vi "GenericDAQCore.vi"(8 "error in":errorcluster, 9 "SignalBuffer queue in":refnum<queue>, 10 "GenericDAQ CtrlQueue in":refnum<queue>) -> (0 "error out":errorcluster)   [LabVIEW 2014, in "GenericDAQ.lvlib"]
uses:
  <instrlib>/GenericDAQ/GenericDAQ.lvlib
  <instrlib>/GenericDAQ/VI/GenericDAQ_Ctrl_Queue.ctl
  <instrlib>/GenericDAQ/VI/GenericDAQ_State.ctl
  <instrlib>/GenericDAQ/VI/GenericDAQ_Signal.ctl
  <instrlib>/GenericDAQ/VI/GenericDAQ_Configs.ctl
  <instrlib>/GenericDAQ/VI/GenericDAQ_PrivateStats.ctl
  <instrlib>/GenericDAQ/VI/GenericDAQ_Status.ctl
  <vilib>/Utility/error.llb/DialogType.ctl
  <instrlib>/GageLv_uic/VI/SetSecondaryDataVIRef_Typedef.ctl
  <vilib>/Utility/error.llb/Error Cluster From Error Code.vi
  <instrlib>/GenericDAQ/VI/InstrParams.vi
  <vilib>/ErrorRing/Error Ring.xnode
  <userlib>/Utility/ErrorLog_lib.lvlib
panel:
  in  "StartAll":bool
  out "Core#":i32
  in  "Get_ConfigAll":bool
  out "LiveStat":T1
  in  "GenericDAQ_Config":T3={"Acquisition"={"Sample Rate"=1000000000.0, "Mode"=0, "Start (0)"=0.0, "Depth"=8192.0, "Segment"=1}, "Channels"=[{"Range"=1, "DC Offset"=0}], "Mode(Gage)"=enum."Continuous"} {"Acquisition"."Depth" min=256.0 step=128.0; "Acquisition"."Mode" items=["Single", "Dual", "Quad", "Octal"]; "Acquisition"."Sample Rate" format="%.0p"}
  out "Graph":sgl[](graph)
  in  "fConfig":bool
  in  "Reset":bool
  in  "CloseAll":bool
  in  "Close":bool
  in  "Enumerate":bool
  in  "Open":bool
  in  "Quit":bool
  in  "Start":bool
  in  "ConfigAll":bool
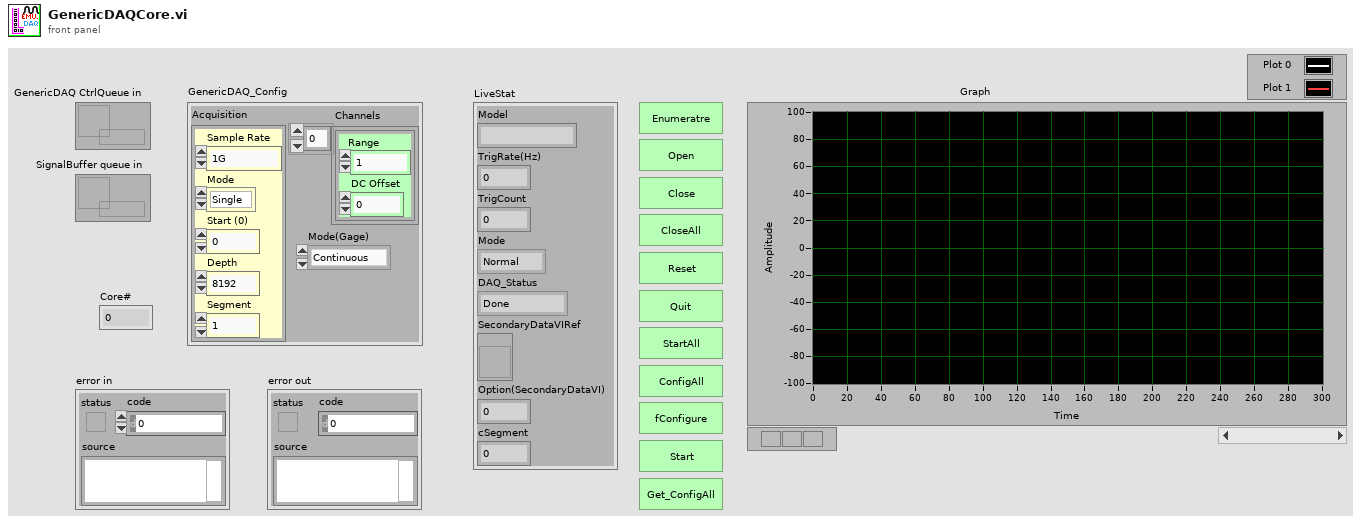
[diagram p1: front panel]
types:
  T1 = typedef "GenericDAQ.lvlib/GenericDAQ_PrivateStats.ctl" = cluster{"Model":string, "TrigRate(Hz)":dbl, "TrigCount":i32, "Mode":enum16{"Normal", "Continuous", "MultiRecord", "HwAverage"}, "DAQ_Status":T2, "SecondaryDataVIRef":refnum<vi>, "Option(SecondaryDataVI)":i32, "cSegment":i32}
  T2 = typedef "GenericDAQ.lvlib/GenericDAQ_Status.ctl" = enum16{"Done", "Armed", "Triggered", "Transfering"}
  T3 = typedef "GenericDAQ.lvlib/GenericDAQ_Configs.ctl" = cluster{"Acquisition":cluster{"Sample Rate":dbl, "Mode":u16, "Start (0)":dbl, "Depth":dbl, "Segment":u32}, "Channels":cluster{"Range":u32, "DC Offset":i32}[], "Mode(Gage)":enum16{"Normal", "Continuous", "MultiRecord", "HwAverage"}}
  T4 = enum16{"Normal", "MultiRecStart", "MultiRecEnd", "Reserved1", "Reserved2", "Reserved3"}
  T5 = typedef "DialogType.ctl" = u16
  T6 = typedef "GenericDAQ.lvlib/GenericDAQ_Signal.ctl" = cluster{"tickcount":u32, "Signal":sgl[], "SecondaryData":dbl[], "Flag":enum16{"Normal", "LineStart", "LineEnd", "FrameStart", "FrameEnd", "Reserved1", "Reserved2"}, "Segment#":i32}
  T7 = enum16{"Normal", "Continuous", "MultiRecord", "HwAverage"}
  T8 = typedef "GenericDAQ.lvlib/GenericDAQ_Ctrl_Queue.ctl" = cluster{"GenericDAQ State":T9, "Variant":variant}
  T9 = typedef "GenericDAQ.lvlib/GenericDAQ_State.ctl" = enum16{"Enumerate", "Open", "Close", "CloseAll", "Reset", "Quit", "==Settings==", "SetAcquisition_", "SetChannels_", "SetTrigger_", "SetAnalogTrigDetector_", "SetSegment#_", "SetAll_AcquChTrig_", "fConfigurate", "fStart", "GetStatus", "_WaitForDone/Idle", "_GetData", "GetAcquisition", "GetChannels", "GetTrigger", "GetAll_AcquChTrig", "Abort", "==Messaging==", "_PushDataOut", "GetStat_", "GetConfig_", "==ModeSetup==", "SetSignalBuffer_", "SetMode_", "SetSecondaryDataRef._", "SetDynamicBuffer_", "==AnalogOut==", "GetChannelCount_AO", "fStart_AO", "SetChEnable_AO", "SetConfig_AO", "SetFuncData_AO", "SetOffset_AO_", "SetMasterNode_AO", "SetStates_AO", "SetSymetry_AO", "SetTriggerSource_AO", "==Trigger==", "ManualTrigger", "===Sync===", "LineStart", "LineEnd", "FrameStart", "FrameEnd", "EOL_PassThrough", "SOL_PassThrough"}
  T10 = typedef "SetSecondaryDataVIRef_Typedef.ctl" = cluster{"SecondaryDataVIRef.":refnum<vi>, "Option":i32}
  T11 = cluster{"Handle":u32, "Sample size":u32, "Resolution":i32, "Offset":i32, "Channels":u32, "Boards":u32}
  T12 = cluster{"Sample Rate":dbl, "Mode":u16, "Start (0)":dbl, "Depth":dbl, "Segment":u32}
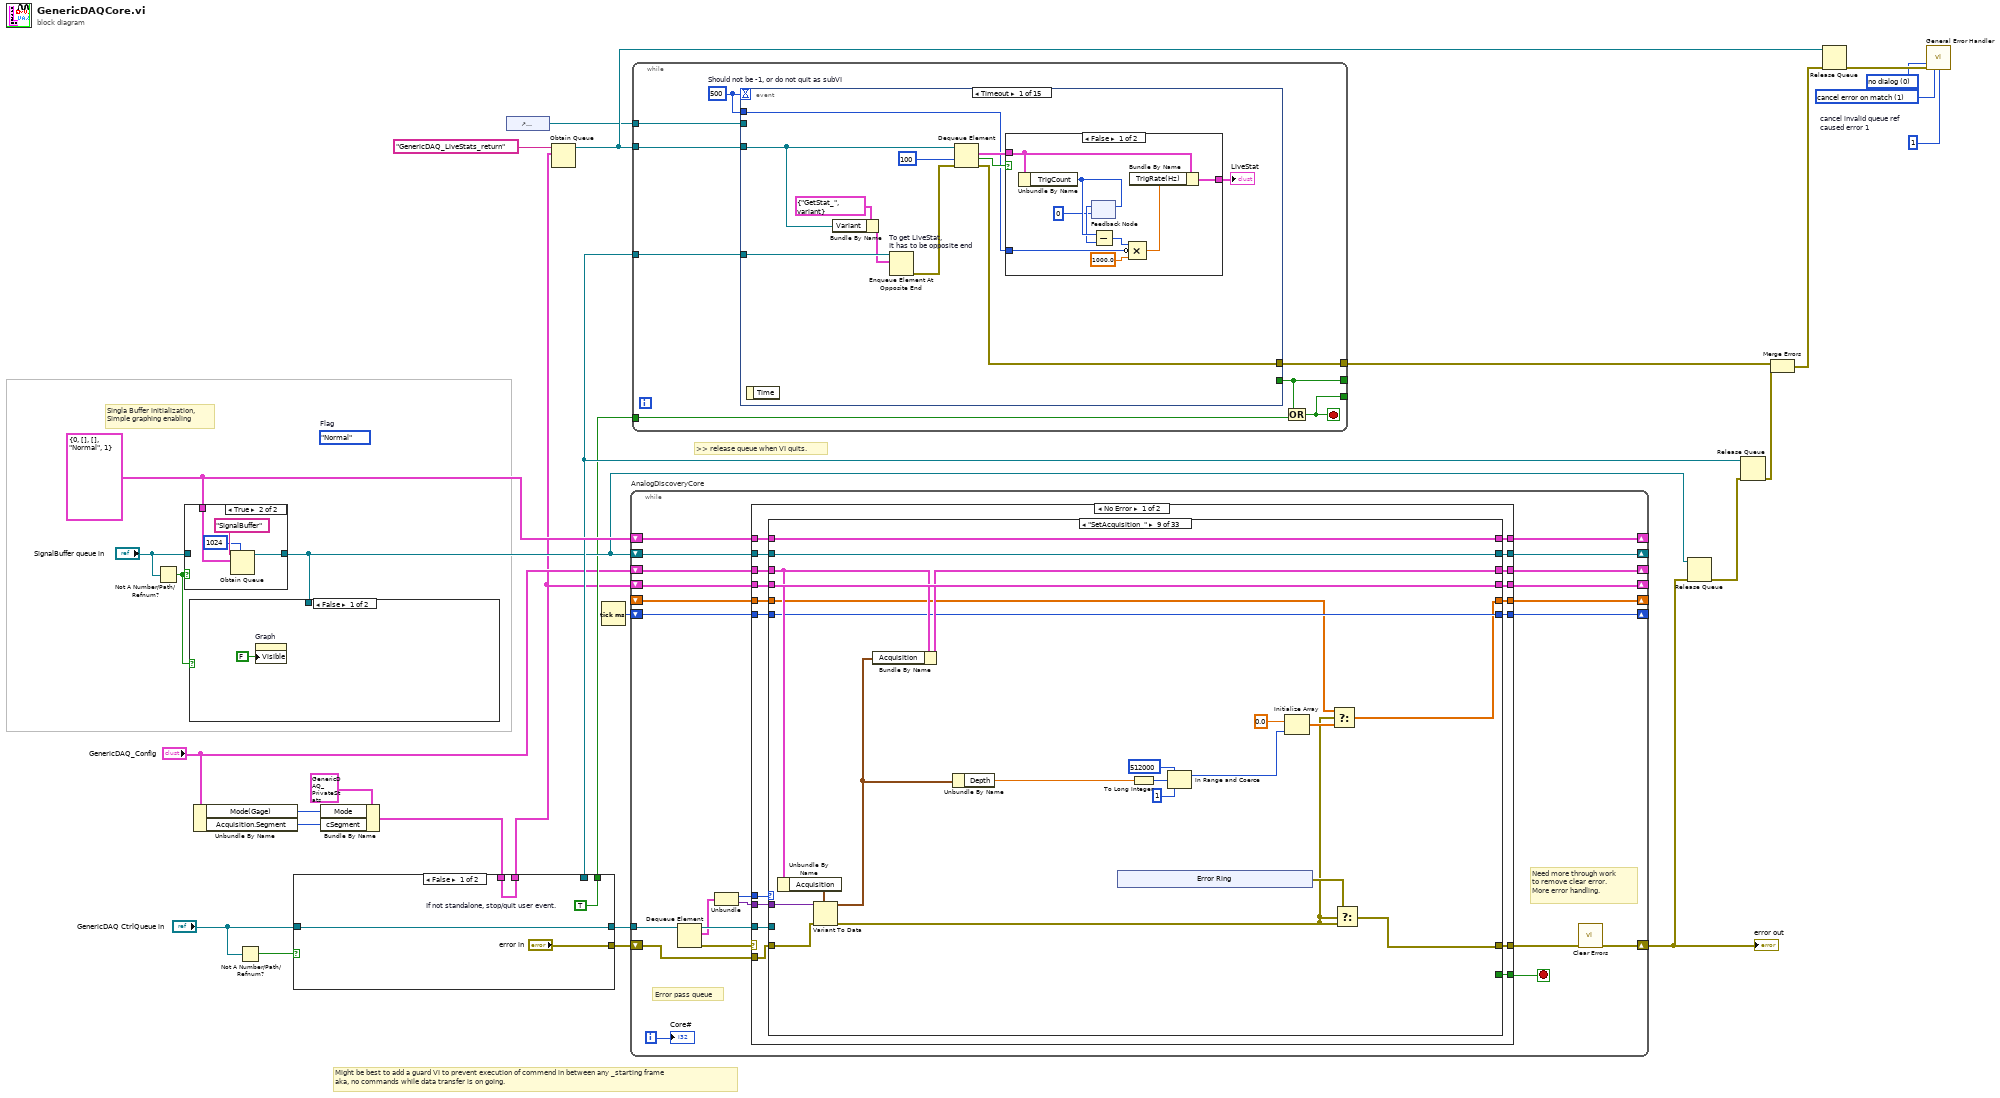
[diagram p0: block diagram]
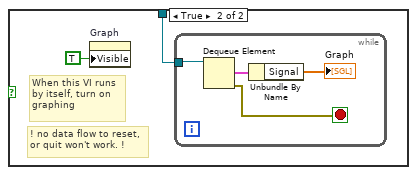
[diagram p2: hidden frame]
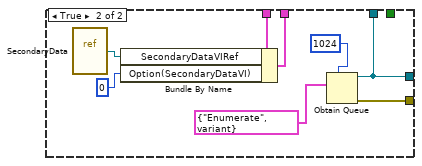
[diagram p4: hidden frame]
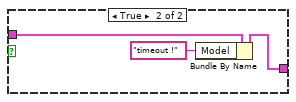
[diagram p5: hidden frame]
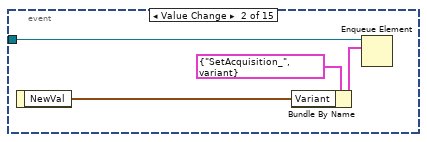
[diagram p6: hidden frame]
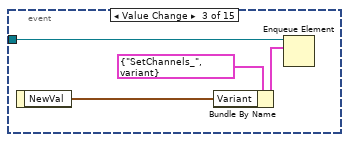
[diagram p7: hidden frame]
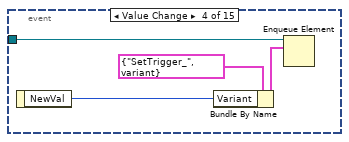
[diagram p8: hidden frame]
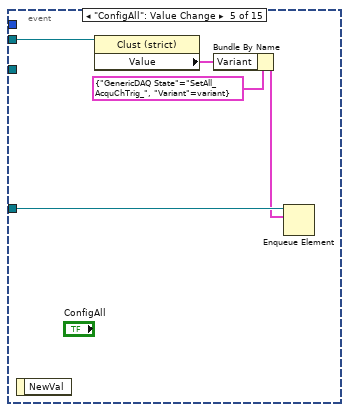
[diagram p9: hidden frame]
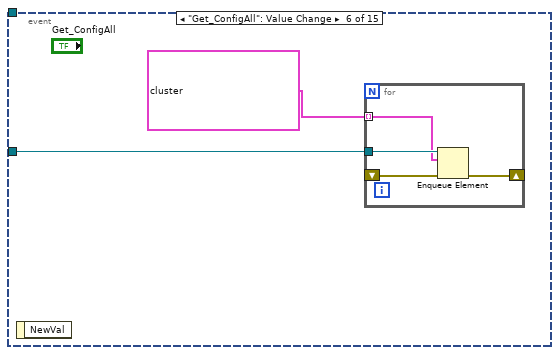
[diagram p10: hidden frame]
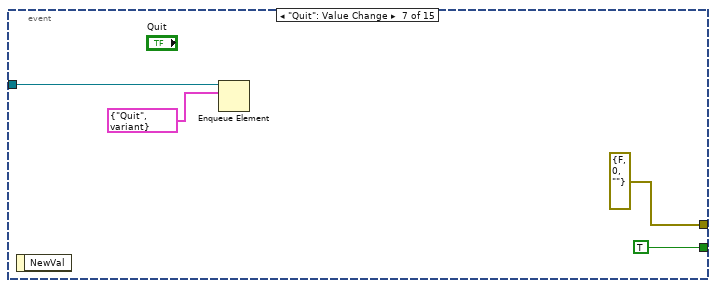
[diagram p11: hidden frame]
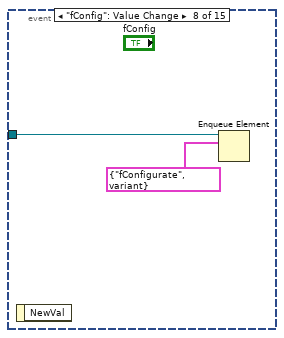
[diagram p12: hidden frame]
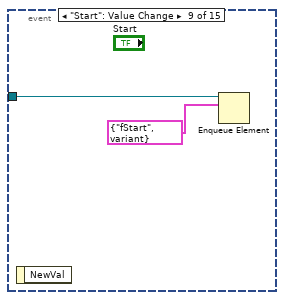
[diagram p13: hidden frame]
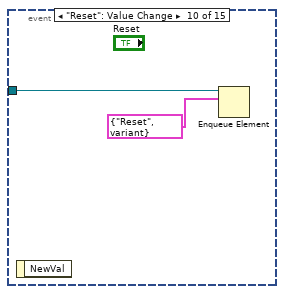
[diagram p14: hidden frame]
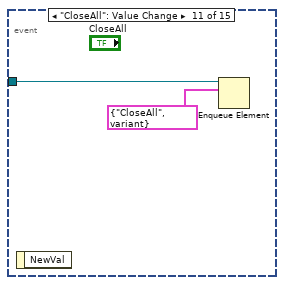
[diagram p15: hidden frame]
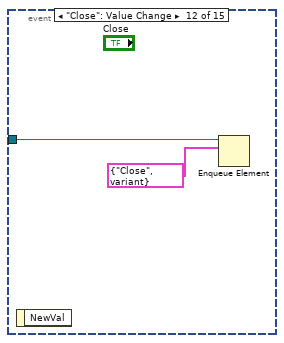
[diagram p16: hidden frame]
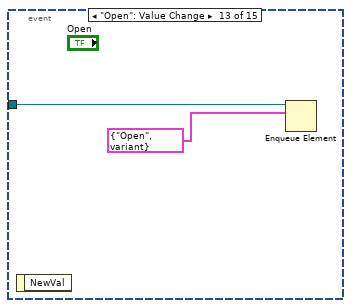
[diagram p17: hidden frame]
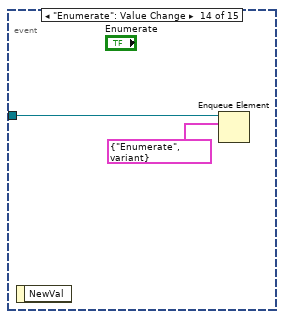
[diagram p18: hidden frame]
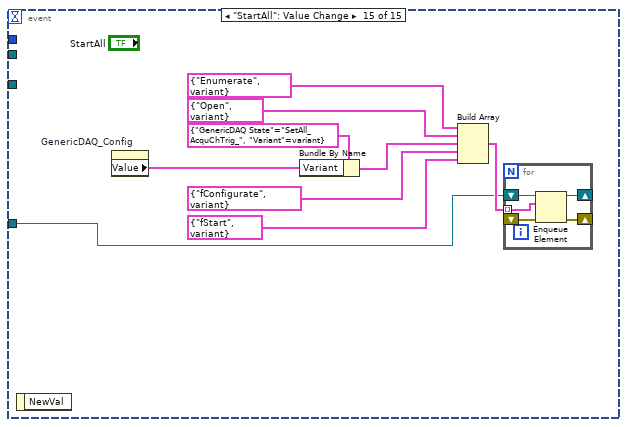
[diagram p19: hidden frame]
diagram:
  (unwired) T4."Normal"  # Flag
  w11 = 1  # cancel invalid queue ref caused error 1
  w12 = 1 items=["no exception", "cancel error on match", "set error on match"] ("[exception action] (none:0)")
  w13 = T5 0 items=["no dialog", "OK message", "continue or stop message", "OK message + warnings", "continue/stop + warnings"] ("type of dialog (OK msg:1)")
  w29 = T6 {"tickcount"=0, "Signal"=[], "SecondaryData"=[], "Flag"=enum."Normal", "Segment#"=1} ("Signal_Typedef")
  # "Might be best to add a guard VI to prevent execution of commend in between any _starting frame \naka, no commands while data transfer is on going."
  # "Singla Buffer initialization,\nSimple graphing enabling"
  # ">> release queue when VI quits."
  n1 = Not A Number/Path/Refnum?(number/path/refnum="SignalBuffer queue in") -> (NaN/Path/Refnum?=w16:bool)
  n2 = case shown="True" w16 {
    tunnel: w29 -> [_ w34]
    tunnel: [w30 w31] -> w17
    tunnel: "SignalBuffer queue in" -> [w30 _]
    frame False {
    }
    frame True {
      n3 = Obtain Queue(max queue size (-1, unlimited)=1024, name (unnamed)="SignalBuffer", element data type=w34) -> (queue out=w31:refnum<queue>)  [unwired: 2 in, 2 out]
    }
  }
  n4 = case shown="False" w16 {
    tunnel: w17 -> [_ w37]
    frame False {
      n5 = property on="Graph" class="WFGraph (strict)"("Visible"=FALSE) -> ()  [unwired: 2 in, 2 out]
    }
    frame True {
      # "! no data flow to reset,\nor quit won't work. !"
      # "When this VI runs\nby itself, turn on \ngraphing"
      n6 = property on="Graph" class="WFGraph (strict)"("Visible"=TRUE) -> ()  [unwired: 2 in, 2 out]
      n7 = while {
        tunnel: w37 -> [w41]
        stop <- w38 stop-if-true
        n8 = Dequeue Element(queue=w41) -> (element=w40:T6, error out=w38:errorcluster)  [unwired: 2 in, 2 out]
        n9 = Unbundle By Name(w40) -> ("Signal"=→"Graph":sgl[])
      }
    }
  }
  n10 = Unbundle By Name("GenericDAQ_Config") -> ("Mode(Gage)"=w7:T7, "Acquisition.Segment"=w4:u32)
  n11 = Not A Number/Path/Refnum?(number/path/refnum="GenericDAQ CtrlQueue in") -> (NaN/Path/Refnum?=w26:bool)
  n12 = Bundle By Name(cluster=T1 {"Model"="", "TrigRate(Hz)"=0.0, "TrigCount"=0, "Mode"=enum."Normal", "DAQ_Status"=enum."Done", "SecondaryDataVIRef"=refnum, "Option(SecondaryDataVI)"=0, "cSegment"=0} ("PrivateStats(Live)"), "Mode"=w7, "cSegment"=w4) -> (w1:T1)
  n13 = case shown="False" w26 {
    tunnel: [w45 w50] -> w28
    tunnel: ["error in" w53] -> w27
    tunnel: "GenericDAQ CtrlQueue in" -> [w45 _]
    tunnel: [_ w50] -> w22
    tunnel: [w43 _] -> w10
    tunnel: [w42 w47] -> w2
    tunnel: w1 -> [w42 w46]
    frame False {
      w43 = TRUE  # If not standalone, stop/quit user event.
    }
    frame True {
      n14 = vi-ref <instrlib>:"SecondaryData.vi"() -> (w49:refnum<vi>)
      n15 = Bundle By Name(cluster=w46, "SecondaryDataVIRef"=w49, "Option(SecondaryDataVI)"=0) -> (w47:T1)
      n16 = Obtain Queue(max queue size (-1, unlimited)=1024, element data type=T8 {"GenericDAQ State"=enum."Enumerate", "Variant"=variant}) -> (queue out=w50:refnum<queue>, error out=w53:errorcluster)  [unwired: 3 in, 1 out]
    }
  }
  n17 = control-ref of="GenericDAQ_Config"() -> (w5:refnum<vi>)
  n18 = Obtain Queue(name (unnamed)="GenericDAQ_LiveStats_return", element data type=w2) -> (queue out=w20:refnum<queue>)  [unwired: 3 in, 2 out]
  n19 = Tick Count (ms)() -> (millisecond timer value=w3:u32)
  n20 = while "AnalogDiscoveryCore" {
    shift-right: [w75] -> _
    shift-left: w17 -> [w76]
    tunnel: w28 -> [w62]
    shift-right: [w56] -> w15
    shift-left: w27 -> [w64]
    shift-right: [w73] -> _
    shift-left: "GenericDAQ_Config" -> [w72]
    shift-right: [w60] -> _
    shift-left: w2 -> [w71]
    shift-right: [w65] -> _
    shift-left: _ -> [w69]
    shift-right: [w66] -> _
    shift-left: w29 -> [w70]
    shift-right: [w54] -> _
    shift-left: w3 -> [w55]
    i -> [w58]
    stop <- w74 stop-if-true
    # "Need more through work\nto remove clear error.\nMore error handling."
    # "Error pass queue"
    n21 = Dequeue Element(queue=w62) -> (queue out=w61:refnum<queue>, element=w59:T8, error out=w63:errorcluster)  [unwired: 2 in, 1 out]
    n22 = Unbundle(w59) -> ("GenericDAQ State"=w68:T9, "Variant"=w67:variant)
    n23 = case shown="No Error" w63 {
      tunnel: w76 -> [w94 w727]
      tunnel: [w93 w727] -> w75
      tunnel: [w92 TRUE] -> w74
      tunnel: [w91 w725] -> w57
      tunnel: [w90 w728] -> w73
      tunnel: w72 -> [w89 w728]
      tunnel: w71 -> [w88 w729]
      tunnel: w70 -> [w87 w726]
      tunnel: w69 -> [w86 w730]
      tunnel: w61 -> [w85 _]
      tunnel: w68 -> [w84 _]
      tunnel: w67 -> [w83 _]
      tunnel: [w82 w726] -> w66
      tunnel: [w81 w730] -> w65
      tunnel: [w80 w729] -> w60
      tunnel: w64 -> [w79 _]
      tunnel: w55 -> [w78 w724]
      tunnel: [w77 w724] -> w54
      frame No Error {
        n24 = case shown="\"SetAcquisition_\"" w84 {
          tunnel: w94 -> [w101 w108 w132 w139 w146 w160 w172 w179 w206 w224 w245 w257 w297 w328 w362 w393 w443 w495 w504 w511 w521 w532 w555 w593 w605 w618 w630 w654 w666 w691 w707 w708 w716]
          tunnel: [w101 w108 w132 w139 w146 w160 w172 w179 w206 w224 w245 w257 w297 w328 w362 w393 w443 w495 w504 w511 w521 w532 w555 w593 w605 w618 w631 w654 w666 w690 w707 w708 w716] -> w93
          tunnel: [_ _ _ _ _ _ TRUE _ _ _ _ _ _ _ _ _ _ _ _ _ _ _ _ _ _ _ _ _ _ _ _ _ _] -> w92
          tunnel: w85 -> [_ _ _ _ _ w156 _ _ _ _ _ w254 w287 w322 _ w395 w439 _ _ _ w516 _ w551 _ _ _ _ _ _ _ _ _ _]
          tunnel: w79 -> [w100 w104 w128 w134 w145 w155 w167 _ w198 w215 _ w248 w288 w319 w358 w394 w437 w494 w503 w510 w515 _ w553 w587 w597 _ w627 w644 _ w694 w706 w715 w723]
          tunnel: [w100 w104 errorcluster {"status"=FALSE, "code"=0, "source"=""} ("error out") w134 w145 w154 w167 w174 w185 w216 errorcluster {"status"=FALSE, "code"=0, "source"=""} ("error out") w253 w286 w323 w358 w388 w440 w494 w503 w510 w514 w527 w552 w586 w598 w613 w628 w645 w656 w694 w706 w715 w723] -> w91
          tunnel: [w99 w107 w131 w138 w144 w159 w171 w178 w203 w221 w241 w251 w296 w327 w361 w392 w445 w490 w500 w509 w517 w531 w549 w585 w595 w617 w636 w653 w665 w700 w705 w714 w722] -> w90
          tunnel: w89 -> [w99 w107 w131 w138 w144 w159 w171 w178 w201 w219 w241 w251 w296 w327 w361 w392 w445 w489 w498 w509 w517 w531 w549 w585 w595 w617 w636 w653 w665 w700 w705 w714 w722]
          tunnel: [w98 w106 w124 w136 w141 w153 w168 w177 w204 w222 w243 w247 w294 w325 w357 w385 w419 w491 w499 w506 w520 w530 w547 w584 w604 w616 w635 w650 w662 w699 w704 w713 w721] -> w80
          tunnel: w88 -> [w98 w106 w129 w136 w141 w153 w168 w177 w204 w222 w243 w247 w294 w325 w356 w386 w434 w491 w499 w506 w520 w530 w548 w584 w604 w616 w635 w649 w657 w699 w704 w713 w721]
          tunnel: w87 -> [w97 w105 w130 w137 w143 w158 w170 w176 w205 w223 w244 w256 w295 w326 w360 w391 w442 w493 w502 w508 w519 w529 w541 w592 w603 w615 w634 w652 w664 w698 w703 w712 w720]
          tunnel: w86 -> [w96 w103 _ w135 w142 w157 w169 w175 w188 w213 w242 w255 w293 w321 w359 w387 w444 w492 w501 w507 w518 w528 w539 w591 w602 w614 w633 w651 w663 w697 w702 w711 w719]
          tunnel: w83 -> [_ _ w127 _ _ _ _ _ w202 w220 _ w252 _ _ _ _ _ _ _ _ _ _ _ w588 w601 _ w632 w648 w660 w695 _ _ _]
          tunnel: [w97 w105 w130 w137 w143 w158 w170 w176 w205 w223 w244 w256 w295 w326 w360 w391 w441 w493 w502 w508 w519 w529 w541 w592 w603 w615 w634 w652 w664 w698 w703 w712 w720] -> w82
          tunnel: [w96 w103 w115 w135 w142 w157 w169 w175 w189 w213 w242 w255 w293 w321 w359 w387 w436 w492 w501 w507 w518 w528 w539 w591 w602 w614 w633 w651 w663 w697 w702 w711 w719] -> w81
          tunnel: w78 -> [w95 w102 w109 w133 w140 w149 w166 w173 w196 w212 w239 w246 w285 w314 w344 w367 w417 w487 w496 w505 w513 w526 w538 w582 w596 w612 w624 w642 w655 w696 w701 w710 w718]
          tunnel: [w95 w102 w109 w133 w140 w149 w166 w173 w196 w212 w239 w246 w285 w314 w344 w370 w417 w487 w496 w505 w513 w526 w538 w582 w596 w612 w624 w642 w655 w696 w701 w710 w718] -> w77
          frame Default {
          }
          frame "Enumerate" {
          }
          frame "Open" {
            (unwired) T11 {"Handle"=0, "Sample size"=1, "Resolution"=256, "Offset"=0, "Channels"=0, "Boards"=0} ("Handle")
            w113 = 8192 ("dimension size")
            w114 = 2 ("16KSa, per spec")
            n25 = Variant To Data(error in=w128, type="", Variant=w127) -> (data=w123:string, error out=w125:errorcluster)
            n26 = Select(t="any", s=TRUE, f=w123) -> (s? t:f=w110:string)
            n27 = Wait (ms)(milliseconds to wait=u32 0) -> ()  [unwired: 1 out]
            n28 = Bundle By Name(cluster=w125, "source"=w110) -> ()  [unwired: 1 out]
            n29 = Bundle By Name(cluster=w129, "Model"=w110, "TrigRate(Hz)"=0.0, "TrigCount"=0) -> (w124:T1)
            n30 = Initialize Array(sgl 0.0 ("Numeric"), w113) -> (w115:sgl[])
            n31 = Initialize Array(i16 0 ("Numeric"), w114, w113) -> ()  [unwired: 1 out]
            n32 = Initialize Array(u8 0 ("Numeric"), w114, w113) -> ()  [unwired: 1 out]
          }
          frame "Close" {
          }
          frame "CloseAll" {
          }
          frame "Reset" {
            n33 = Unbundle By Name(w153) -> ("Model"=w152:string)
            n34 = Bundle By Name(cluster=T8 {"GenericDAQ State"=enum."Open", "Variant"=variant} ("element"), "Variant"=w152) -> (w151:T8)
            n35 = Build Array(w151, T8 {"GenericDAQ State"=enum."Close", "Variant"=variant} ("element")) -> (w150:T8[])
            n36 = for {
              tunnel: w156 -> [w164]
              tunnel: w150 -> [w161] mode=indexing
              shift-right: [w162] -> w154
              shift-left: w155 -> [w163]
              n37 = Enqueue Element At Opposite End(queue=w164, element=w161, error in (no error)=w163) -> (error out=w162:errorcluster)  [unwired: 1 in, 2 out]
            }
          }
          frame "Quit" {
          }
          frame "==Settings==" {
            # "Invalid frame"
            n38 = xnode "Error Ring"() -> ("error out"=w174:errorcluster)
          }
          frame "SetAcquisition_" {
            n39 = Unbundle By Name(w201) -> ("Acquisition"=w200:T12)
            n40 = Variant To Data(error in=w198, type=w200, Variant=w202) -> (data=w199:T12, error out=w186:errorcluster)
            n41 = Bundle By Name(cluster=w201, "Acquisition"=w199) -> (w203:T3)
            n42 = Unbundle By Name(w199) -> ("Depth"=w192:dbl)
            n43 = xnode "Error Ring"() -> ("error out"=w187:errorcluster)
            n44 = To Long Integer(number=w192) -> (32bit integer=w191:i32)
            n45 = In Range and Coerce(upper limit=512000, x=w191, lower limit=1) -> (coerced(x)=w190:i32)  [unwired: 1 out]
            n46 = Initialize Array(sgl 0.0 ("Numeric"), w190) -> (w197:sgl[])
            n47 = Select(t=w188, s=w186, f=w197) -> (s? t:f=w189:sgl[])
            n48 = Select(t=w187, s=w186, f=w186) -> (s? t:f=w185:errorcluster)
          }
          frame "SetChannels_" {
            n49 = Unbundle By Name(w219) -> ("Channels"=w218:cluster{"Range":u32, "DC Offset":i32}[])
            n50 = Variant To Data(error in=w215, type=w218, Variant=w220) -> (data=w217:cluster{"Range":u32, "DC Offset":i32}[], error out=w214:errorcluster)
            n51 = Bundle By Name(cluster=w219, "Channels"=w217) -> (w221:T3)
            n52 = case shown="No Error" w214 {
              selector: w214 -> [w225 _]
              tunnel: w222 -> [_ _]
              tunnel: w217 -> [w227 _]
              tunnel: [w226 w233] -> w216
              frame No Error {
                n53 = for {
                  tunnel: w227 -> [w229] mode=indexing
                  shift-right: [w232] -> w226
                  shift-left: w225 -> [w232]
                  tunnel: [w228] -> _ mode=indexing
                  n54 = Unbundle By Name(w229) -> ("Range"=w230:u32, "DC Offset"=w231:i32)
                  n55 = Bundle("Range"=w230, "DC Offset"=w231) -> (w228:cluster{"Range":u32, "DC Offset":i32})  [unwired: 1 in]
                }
              }
              frame Error {
                n56 = xnode "Error Ring"() -> ("error out"=w233:errorcluster)
              }
            }
          }
          frame "SetTrigger_" {
          }
          frame "SetAll_AcquChTrig_" {
            n57 = Variant To Data(type=w251, Variant=w252) -> (data=w249:T3, error out=w250:errorcluster)  [unwired: 1 in]
            n58 = case shown="No Error" w250 {
              tunnel: w254 -> [w273 _]
              tunnel: [w272 w278] -> w253
              tunnel: w249 -> [w271 _]
              tunnel: w248 -> [w270 _]
              frame No Error {
                n59 = Unbundle By Name(w271) -> ("Mode(Gage)"=w262:T7, "Acquisition"=w268:T12, "Channels"=w266:cluster{"Range":u32, "DC Offset":i32}[])
                n60 = Bundle By Name(cluster=T8 {"GenericDAQ State"=enum."SetMode_", "Variant"=variant} ("element"), "Variant"=w262) -> (w259:T8)
                n61 = Bundle By Name(cluster=T8 {"GenericDAQ State"=enum."SetAcquisition_", "Variant"=variant} ("element"), "Variant"=w268) -> (w260:T8)
                n62 = Bundle By Name(cluster=T8 {"GenericDAQ State"=enum."SetChannels_", "Variant"=variant} ("element"), "Variant"=w266) -> (w258:T8)
                n63 = Build Array(w259, w260, w258, T8 {"GenericDAQ State"=enum."SetTrigger_", "Variant"=variant} ("element")) -> (w264:T8[])
                n64 = Reverse 1D Array(array=w264) -> (reversed array=w261:T8[])
                n65 = for "Has to be at the \nopposite end, otherwise\nrace condition" {
                  tunnel: w273 -> [w277]
                  shift-right: [w276] -> w272
                  shift-left: w270 -> [w275]
                  tunnel: w261 -> [w274] mode=indexing
                  n66 = Enqueue Element At Opposite End(queue=w277, element=w274, error in (no error)=w275) -> (error out=w276:errorcluster)  [unwired: 1 in, 2 out]
                }
              }
              frame Error {
                n67 = xnode "Error Ring"() -> ("error out"=w278:errorcluster)
              }
            }
          }
          frame "fConfigurate" {
            # "If dependancy of ErrorLog missing, \njust remove errorlog vi."
            n68 = Flush Queue(queue=w287, error in (no error)=w288) -> (queue out=w292:refnum<queue>, remaining elements=w290:T8[], error out=w291:errorcluster)
            n69 = for "Remove unfinished acquisition process" {
              shift-right: [w304] -> _
              shift-left: w292 -> [w305]
              shift-right: [w302] -> w289
              shift-left: w291 -> [w303]
              tunnel: w290 -> [w298] mode=indexing
              tunnel: T8[] [{"GenericDAQ State"=enum."_WaitForDone/Idle", "Variant"=variant}, {"GenericDAQ State"=enum."_GetData", "Variant"=variant}, {"GenericDAQ State"=enum."_PushDataOut", "Variant"=variant}] -> [w301]
              n70 = Search 1D Array(1D array=w301, element=w298) -> (index of element=w300:i32)  [unwired: 1 in]
              n71 = Greater Or Equal To 0?(x=w300) -> (x >= 0?=w299:bool)
              n72 = case shown="False" w299 {
                tunnel: w305 -> [w310 w312]
                tunnel: [w309 w312] -> w304
                tunnel: w303 -> [w308 w311]
                tunnel: [w307 w311] -> w302
                tunnel: w298 -> [w306 _]
                frame False {
                  n73 = Enqueue Element(queue=w310, element=w306, error in (no error)=w308) -> (queue out=w309:refnum<queue>, error out=w307:errorcluster)  [unwired: 1 in, 1 out]
                }
                frame True {
                }
              }
            }
            n74 = call <userlib>:"ErrorLog.vi"("error in (no error)"=w289) -> ("error out"=w286:errorcluster)  [unwired: 10 in]
          }
          frame "fStart" {
            n75 = Flush Queue(queue=w322, error in (no error)=w319) -> (queue out=w320:refnum<queue>, remaining elements=w315:T8[], error out=w317:errorcluster)
            n76 = for "Remove unfinished acquisition process" {
              shift-right: [w335] -> w318
              shift-left: w320 -> [w336]
              shift-right: [w333] -> w316
              shift-left: w317 -> [w334]
              tunnel: w315 -> [w329] mode=indexing
              tunnel: T8[] [{"GenericDAQ State"=enum."_WaitForDone/Idle", "Variant"=variant}, {"GenericDAQ State"=enum."_GetData", "Variant"=variant}, {"GenericDAQ State"=enum."_PushDataOut", "Variant"=variant}] -> [w332]
              n77 = Search 1D Array(1D array=w332, element=w329) -> (index of element=w331:i32)  [unwired: 1 in]
              n78 = Greater Or Equal To 0?(x=w331) -> (x >= 0?=w330:bool)
              n79 = case shown="False" w330 {
                tunnel: w336 -> [w341 w343]
                tunnel: [w340 w343] -> w335
                tunnel: w334 -> [w339 w342]
                tunnel: [w338 w342] -> w333
                tunnel: w329 -> [w337 _]
                frame False {
                  n80 = Enqueue Element(queue=w341, element=w337, error in (no error)=w339) -> (queue out=w340:refnum<queue>, error out=w338:errorcluster)  [unwired: 1 in, 1 out]
                }
                frame True {
                }
              }
            }
            n81 = Enqueue Element(queue=w318, element=T8 {"GenericDAQ State"=enum."_WaitForDone/Idle", "Variant"=variant}, error in (no error)=w316) -> (error out=w323:errorcluster)  [unwired: 1 in, 2 out]
          }
          frame "GetStatus" {
            n82 = Tick Count (ms)() -> (millisecond timer value=w345:u32)
            n83 = Quotient & Remainder(x=u32 1000, y=u32 500) -> (floor(x/y)=w350:u32)  [unwired: 1 out]
            n84 = Subtract(x=w345, y=w344) -> (x-y=w351:u32)
            n85 = Greater?(x=w351, y=w350) -> (0:w349:bool)
            n86 = And(x=w349, y=TRUE) -> (x .and. y?=w347:bool)
            n87 = Select(t=GenericDAQ_Status."Done" ("DAQ_Status"), s=w347, f=GenericDAQ_Status."Armed" ("DAQ_Status")) -> (s? t:f=w348:T2)
            n88 = Bundle By Name(cluster=w356, "DAQ_Status"=w348) -> (w357:T1)
          }
          frame "_WaitForDone/Idle" {
            w365 = T9[] [enum."Close", enum."CloseAll", enum."Reset", enum."Quit"] items=["Enumerate", "Open", "Close", "CloseAll", "Reset", "Quit", "==Settings==", "SetAcquisition_", "SetChannels_", "SetTrigger_", "SetAnalogTrigDetector_", "SetSegment#_", "SetAll_AcquChTrig_", "fConfigurate", "fStart", "GetStatus", "_WaitForDone/Idle", "_GetData", "GetAcquisition", "GetChannels", "GetTrigger", "GetAll_AcquChTrig", "Abort", "==Messaging==", "_PushDataOut", "GetStat_", "GetConfig_", "==ModeSetup==", "SetSignalBuffer_", "SetMode_", "SetSecondaryDataRef._", "SetDynamicBuffer_", "==AnalogOut==", "GetChannelCount_AO", "fStart_AO", "SetChEnable_AO", "SetConfig_AO", "SetFuncData_AO", "SetOffset_AO_", "SetMasterNode_AO", "SetStates_AO", "SetSymetry_AO", "SetTriggerSource_AO", "==Trigger==", "ManualTrigger", "===Sync===", "LineStart", "LineEnd", "FrameStart", "FrameEnd", "EOL_PassThrough", "SOL_PassThrough"]
            # "Simulate repetition rate"
            # "0 dne\n1 armed\n2 triggered\n3 transfering"
            n89 = global read "InstrParams.vi" "TriggerRate"() -> (w363:u32)
            n90 = Tick Count (ms)() -> (millisecond timer value=w369:u32)
            n91 = Wait Until Next ms Multiple(millisecond multiple=u32 0 ("milliseconds to wait")) -> ()  [unwired: 1 out]
            n92 = global read "InstrParams.vi" "SignalOn"() -> (w364:bool)
            n93 = Quotient & Remainder(x=u32 1000, y=w363) -> (floor(x/y)=w372:u32)  [unwired: 1 out]
            n94 = Subtract(x=w369, y=w367) -> (x-y=w373:u32)
            n95 = Greater Or Equal?(x=w373, y=w372) -> (x >= y?=w371:bool)
            n96 = And(x=w371, y=w364) -> (x .and. y?=w368:bool)
            n97 = Preview Queue Element(queue=w395, timeout in ms (-1)=0, error in (no error)=w394) -> (queue out=w390:refnum<queue>, element=w383:T8, timed out?=w382:bool, error out=w389:errorcluster)
            n98 = Unbundle(w383) -> ("GenericDAQ State"=w379:T9)  [unwired: 1 out]
            n99 = Select(t=GenericDAQ_Status."Done" ("DAQ_Status"), s=w368, f=GenericDAQ_Status."Armed" ("DAQ_Status")) -> (s? t:f=w366:T2)
            n100 = Select(t=w369, s=w368, f=w367) -> (s? t:f=w370:u32)
            n101 = Search 1D Array(1D array=w365, element=w379) -> (index of element=w381:i32)  [unwired: 1 in]
            n102 = Greater Or Equal To 0?(x=w381) -> (x >= 0?=w380:bool)
            n103 = Bundle By Name(cluster=w386, "DAQ_Status"=w366) -> (w385:T1)
            n104 = Compound Arithmetic op=AND(w380, invert w382) -> (w378:bool)
            n105 = case shown="False" w378 {
              tunnel: w390 -> [w399 _]
              tunnel: w389 -> [w398 w416]
              tunnel: [w397 w416] -> w388
              tunnel: w366 -> [w396 _]
              frame False {
                n106 = case shown="\"Done\"" w396 {
                  tunnel: w399 -> [w400 w411 w415]
                  tunnel: w398 -> [w403 w410 w414]
                  tunnel: [w402 w409 w413] -> w397
                  frame "Armed" {
                    # "armed ??"
                    # "Typically, this is caused by config change\nduring acquisition. \nPush fConfig and fStart to continure  acuisition."
                    # "armed, not configed??"
                    n107 = for {
                      shift-right: [w406] -> w402
                      shift-left: w403 -> [w407]
                      tunnel: T8[] [{"GenericDAQ State"=enum."_WaitForDone/Idle", "Variant"=variant}] -> [w405] mode=indexing
                      tunnel: w400 -> [w404]
                      n108 = Enqueue Element(queue=w404, element=w405, error in (no error)=w407) -> (error out=w406:errorcluster)  [unwired: 1 in, 2 out]
                    }
                  }
                  frame "Done" {
                    # "Done"
                    n109 = Enqueue Element(queue=w411, element=T8 {"GenericDAQ State"=enum."_GetData", "Variant"=variant}, error in (no error)=w410) -> (error out=w409:errorcluster)  [unwired: 1 in, 2 out]
                  }
                  frame "Triggered", Default {
                    # "triggered"
                    # "triggered, others"
                    n110 = Enqueue Element(queue=w415, element=T8 {"GenericDAQ State"=enum."_WaitForDone/Idle", "Variant"=variant}, error in (no error)=w414) -> (error out=w413:errorcluster)  [unwired: 1 in, 2 out]
                  }
                }
              }
              frame True {
              }
            }
          }
          frame "_GetData" {
            n111 = Unbundle By Name(w445) -> ("Acquisition.Segment"=w423:u32, "Channels"=w432:cluster{"Range":u32, "DC Offset":i32}[], "Acquisition.Depth"=w431:dbl, "Acquisition.Start (0)"=w428:dbl)
            n112 = Unbundle By Name(w434) -> ("TrigCount"=w433:i32, "Option(SecondaryDataVI)"=w427:i32, "SecondaryDataVIRef"=w418:refnum<vi>, "cSegment"=w421:i32)
            n113 = Unbundle By Name(w434) -> ("Mode"=w424:T7)
            n114 = Enqueue Element(queue=w439, element=T8 {"GenericDAQ State"=enum."_PushDataOut", "Variant"=variant}, error in (no error)=w437) -> (error out=w429:errorcluster)  [unwired: 1 in, 2 out]
            n115 = Array Size(array=w432) -> (size(s)=w430:i32)
            n116 = Decrement(x=w421) -> (x-1=w422:i32)
            n117 = Subtract(x=w423, y=w422) -> (x-y=w425:u32)
            n118 = for {
              N: w430 -> [_]
              tunnel: w444 -> [w485]
              tunnel: [w484] -> w436 mode=concatenating
              tunnel: w431 -> [_]
              tunnel: w428 -> [_]
              shift-right: [w486] -> w426
              shift-left: w429 -> [w486]
              tunnel: w425 -> [_]
              tunnel: w418 -> [w483]
              n119 = call <instrlib>:"GenerateFakeSignal.vi"("SecondaryDataVIRef"=w483, "Array"=w485) -> ("simulated signal"=w484:sgl[])  [unwired: 9 in]
            }
            n120 = Increment(x=w433) -> (x+1=w435:i32)
            n121 = Bundle By Name(cluster=w434, "TrigCount"=w435, "cSegment"=w422) -> (w420:T1)
            n122 = case shown="\"Continuous\", Default" w424 {
              tunnel: w442 -> [w454 w466 w479]
              tunnel: [w453 w466 w478] -> w441
              tunnel: [w449 w465 w474] -> w440
              tunnel: w418 -> [w452 _ w477]
              tunnel: w427 -> [w451 _ w476]
              tunnel: w426 -> [w449 w464 w474]
              tunnel: w422 -> [_ w460 _]
              tunnel: w423 -> [_ w458 _]
              tunnel: w420 -> [w446 w462 w471]
              tunnel: [w446 w461 w471] -> w419
              frame "Continuous", Default {
                n123 = Not A Number/Path/Refnum?(number/path/refnum=w452) -> (NaN/Path/Refnum?=w447:bool)
                n124 = case shown="False" w447 {
                  tunnel: [w457 _] -> w448
                  tunnel: w452 -> [w456 _]
                  tunnel: w451 -> [w455 _]
                  frame False {
                    n125 = call-by-ref "?"(reference=w456, "Option"=w455) -> ("SecondaryData"=w457:dbl[])  [unwired: 11 in, 2 out]
                  }
                  frame True {
                  }
                }
                n126 = Tick Count (ms)() -> (millisecond timer value=w450:u32)
                n127 = Bundle By Name(cluster=w454, "tickcount"=w450, "SecondaryData"=w448) -> (w453:T6)
              }
              frame "MultiRecord" {
                n128 = Increment(x=w460) -> (x+1=w459:i32)
                n129 = case shown="0" w460 {
                  tunnel: [w469 w470] -> w465
                  tunnel: w464 -> [w469 w470]
                  frame 0 {
                    # "End of MultiRecord Transfer, start next"
                  }
                  frame Default {
                  }
                }
                n130 = Equal?(x=w458, y=w459) -> (x = y?=w463:bool)
                n131 = case shown="True" w463 {
                  tunnel: w459 -> [_ _]
                  tunnel: w462 -> [w467 w468]
                  tunnel: [w467 w468] -> w461
                  frame False {
                  }
                  frame True {
                    # "Get TS array at the first record"
                  }
                }
              }
              frame "Normal" {
                n132 = Not A Number/Path/Refnum?(number/path/refnum=w477) -> (NaN/Path/Refnum?=w472:bool)
                n133 = case shown="False" w472 {
                  tunnel: [w482 _] -> w473
                  tunnel: w477 -> [w481 _]
                  tunnel: w476 -> [w480 _]
                  frame False {
                    n134 = call-by-ref "?"(reference=w481, "Option"=w480) -> ("SecondaryData"=w482:dbl[])  [unwired: 11 in, 2 out]
                  }
                  frame True {
                  }
                }
                n135 = Tick Count (ms)() -> (millisecond timer value=w475:u32)
                n136 = Bundle By Name(cluster=w479, "tickcount"=w475, "SecondaryData"=w473) -> (w478:T6)
              }
            }
          }
          frame "GetAcquisition" {
            n137 = Unbundle By Name(w489) -> ("Acquisition.Sample Rate"=w488:dbl)
            n138 = Bundle By Name(cluster=w489, "Acquisition.Sample Rate"=w488) -> (w490:T3)
          }
          frame "GetChannels" {
            n139 = Unbundle By Name(w498) -> ("Channels"=w497:cluster{"Range":u32, "DC Offset":i32}[])
            n140 = Bundle By Name(cluster=w498, "Channels"=w497) -> (w500:T3)
          }
          frame "GetTrigger" {
          }
          frame "GetAll_AcquChTrig" {
            n141 = for "Has to be at the \nopposite end, otherwise\nrace condition" {
              tunnel: w516 -> [w525]
              shift-right: [w524] -> w514
              shift-left: w515 -> [w523]
              tunnel: T8[] [{"GenericDAQ State"=enum."GetAcquisition", "Variant"=variant}, {"GenericDAQ State"=enum."GetChannels", "Variant"=variant}, {"GenericDAQ State"=enum."GetTrigger", "Variant"=variant}] -> [w522] mode=indexing
              n142 = Enqueue Element At Opposite End(queue=w525, element=w522, error in (no error)=w523) -> (error out=w524:errorcluster)  [unwired: 1 in, 2 out]
            }
          }
          frame "==Messaging==" {
            # "Invalid Frame"
            n143 = xnode "Error Ring"() -> ("error out"=w527:errorcluster)
          }
          frame "_PushDataOut" {
            n144 = Unbundle By Name(w549) -> ("Acquisition.Segment"=w546:u32)  [unwired: 1 out]
            n145 = Unbundle By Name(w548) -> ("Mode"=w554:T7)
            n146 = Unbundle By Name(w548) -> ("cSegment"=w545:i32)
            n147 = case shown="\"MultiRecord\"" w554 {
              tunnel: w553 -> [w557 w564 w581]
              tunnel: [w557 w563 w580] -> w552
              tunnel: w551 -> [_ w562 w579]
              tunnel: w548 -> [w556 w560 w578]
              tunnel: [w556 w559 w577] -> w547
              tunnel: w546 -> [_ w558 w569]
              tunnel: w545 -> [_ _ w568]
              tunnel: [_ _ TRUE] -> w543
              tunnel: [_ _ u32 0 ("unsigned 32bit integer")] -> w540
              frame "Normal" {
              }
              frame "Continuous", Default {
                # "In continuous single trigger  mode, \nre-arming is done in \"_GetData\"\n\nNormal mode => no need to re-arming  daq"
                n148 = Enqueue Element(queue=w562, element=T8 {"GenericDAQ State"=enum."_WaitForDone/Idle", "Variant"=variant}, error in (no error)=w564) -> (error out=w563:errorcluster)  [unwired: 1 in, 2 out]
                n149 = Bundle By Name(cluster=w560, "cSegment"=w558) -> (w559:T1)
              }
              frame "MultiRecord" {
                w565 = 1000.0 ("y")
                # "3 functions:\n1. retrival of timestamp\n2. reset cSegment counter\n3. decide continue transfer or wait for next round"
                n150 = Subtract(x=w569, y=w568) -> (x-y=w570:u32)
                n151 = Equal To 0?(x=w568) -> (x = 0?=w575:bool)
                n152 = Decrement "Get Index"(x=w570) -> ()  [unwired: 1 out]
                n153 = Select(t=w569, s=w575, f=w568) -> (s? t:f=w576:u32)
                n154 = Select(t=T8 {"GenericDAQ State"=enum."_WaitForDone/Idle", "Variant"=variant} ("element"), s=w575, f=T8 {"GenericDAQ State"=enum."_GetData", "Variant"=variant} ("element")) -> (s? t:f=w572:T8)
                n155 = Multiply(x=w565, y=w565) -> (x*y=w567:dbl)
                n156 = Bundle By Name(cluster=w578, "cSegment"=w576) -> (w577:T1)
                n157 = Enqueue Element(queue=w579, element=w572, error in (no error)=w581) -> (error out=w580:errorcluster)  [unwired: 1 in, 2 out]
                n158 = To Unsigned Long Integer(number=w567) -> ()  [unwired: 1 out]
              }
            }
            n159 = Unbundle By Name(w541) -> ("tickcount"=w542:u32)
            n160 = Select(t=w540, s=w543, f=w542) -> (s? t:f=w544:u32)
            n161 = Bundle By Name(cluster=w541, "Signal"=w539, "tickcount"=w544) -> (w550:T6)
            n162 = Enqueue Element "Send/Push Data Out"(queue=w555, element=w550) -> ()  [unwired: 2 in, 3 out]
          }
          frame "GetStat_" {
            n163 = Variant To Data(error in=w587, type=refnum<queue> refnum ("queue out"), Variant=w588) -> (data=w590:refnum<queue>, error out=w589:errorcluster)
            n164 = Enqueue Element "Send Core Stat"(queue=w590, element=w584, error in (no error)=w589) -> (error out=w586:errorcluster)  [unwired: 1 in, 2 out]
          }
          frame "GetConfig_" {
            n165 = Variant To Data(type=refnum<queue> refnum ("queue out"), Variant=w601) -> (data=w600:refnum<queue>, error out=w599:errorcluster)  [unwired: 1 in]
            n166 = case shown="No Error" w599 {
              selector: w599 -> [_ w611]
              tunnel: w600 -> [w609 _]
              tunnel: w595 -> [w606 _]
              tunnel: [w608 w611] -> w598
              tunnel: w597 -> [w607 _]
              frame No Error {
                n167 = Enqueue Element(queue=w609, element=w606, error in (no error)=w607) -> (error out=w608:errorcluster)  [unwired: 1 in, 2 out]
              }
              frame Error {
                n168 = One Button Dialog(message="Internal error in \"GetConfig_\"\nWrong type for querystatus.\nNo response sent, outer loop will wait forever.\nCheck caller syntax to fix it. ") -> ()  [unwired: 1 in, 1 out]
              }
            }
          }
          frame "==ModeSetup==" {
            n169 = xnode "Error Ring"() -> ("error out"=w613:errorcluster)
          }
          frame "SetSignalBuffer_" {
            n170 = Variant To Data(type=w630, Variant=w632) -> (data=w629:refnum<queue>, error out=w626:errorcluster)  [unwired: 1 in]
            n171 = Select(t=w630, s=w626, f=w629) -> (s? t:f=w631:refnum<queue>)
            n172 = xnode "Error Ring"() -> ("error out"=w625:errorcluster)
            n173 = Select(t=w625, s=w626, f=w627) -> (s? t:f=w628:errorcluster)
          }
          frame "SetMode_" {
            n174 = Unbundle By Name(w649) -> ("Mode"=w647:T7)
            n175 = Variant To Data(error in=w644, type=w647, Variant=w648) -> (data=w646:T7, error out=w645:errorcluster)
            n176 = Select(t=w647, s=w645, f=w646) -> (s? t:f=w643:T7)
            n177 = Bundle By Name(cluster=w649, "Mode"=w643) -> (w650:T1)
          }
          frame "SetSecondaryDataRef._" {
            n178 = Variant To Data(type=T10 {"SecondaryDataVIRef."=refnum, "Option"=0} ("SecondaryDataParams."), Variant=w660) -> (data=w658:T10, error out=w659:errorcluster)  [unwired: 1 in]
            n179 = case shown="No Error" w659 {
              tunnel: w657 -> [w680 w684]
              tunnel: [w679 w684] -> w662
              tunnel: w658 -> [w675 _]
              tunnel: w657 -> [w672 _]
              tunnel: [w667 w683] -> w656
              frame No Error {
                n180 = Unbundle By Name(w672) -> ("SecondaryDataVIRef"=w670:refnum<vi>)
                n181 = Unbundle By Name(w675) -> ("SecondaryDataVIRef."=w674:refnum<vi>, "Option"=w673:i32)
                n182 = Not A Number/Path/Refnum?(number/path/refnum=w670) -> (NaN/Path/Refnum?=w671:bool)
                n183 = case shown="False" w671 {
                  tunnel: w670 -> [w682 _]
                  tunnel: [w681 _] -> w669
                  frame False {
                    n184 = Close Reference(reference=w682) -> (error out=w681:errorcluster)  [unwired: 1 in]
                  }
                  frame True {
                  }
                }
                n185 = property class="VI Interface Type 1"(reference=w674, error in=w669) -> (reference out=w677:refnum<vi>, error out=w668:errorcluster, "Path"=w678:path)
                n186 = Open VI Reference(type specifier VI Refnum (for type only)=w677, vi path=w678, error in (no error)=w668) -> (vi reference=w676:refnum<vi>, error out=w667:errorcluster)  [unwired: 3 in]
                n187 = Bundle By Name(cluster=w680, "SecondaryDataVIRef"=w676, "Option(SecondaryDataVI)"=w673) -> (w679:T1)
              }
              frame Error {
                n188 = xnode "Error Ring"() -> ("error out"=w683:errorcluster)
              }
            }
          }
          frame "SetDynamicBuffer_" {
            n189 = Variant To Data(error in=w694, type=w691, Variant=w695) -> (data=w692:refnum<queue>, error out=w693:errorcluster)
            n190 = Select(t=w691, s=w693, f=w692) -> (s? t:f=w690:refnum<queue>)
          }
          frame "===Sync===" {
          }
          frame "LineStart", "SOL_PassThrough" {
            n191 = Enqueue Element(queue=w708, element=T6 {"tickcount"=0, "Signal"=[], "SecondaryData"=[], "Flag"=enum."LineStart", "Segment#"=0}) -> ()  [unwired: 2 in, 3 out]
          }
          frame "LineEnd", "EOL_PassThrough" {
            n192 = Enqueue Element(queue=w716, element=T6 {"tickcount"=0, "Signal"=[], "SecondaryData"=[], "Flag"=enum."LineEnd", "Segment#"=0}) -> ()  [unwired: 2 in, 3 out]
          }
        }
      }
      frame Error {
        n193 = xnode "Error Ring"() -> ("error out"=w725:errorcluster)
      }
    }
    n194 = call <vilib>:"Clear Errors.vi"("error in (no error)"=w57) -> ("error out"=w56:errorcluster)  [unwired: 5 in, 1 out]
    "Core#" <- w58
  }
  "error out" <- w15
  n195 = while {
    tunnel: w22 -> [w744]
    tunnel: w5 -> [w743]
    tunnel: w20 -> [w742]
    tunnel: w10 -> [w741]
    tunnel: [w740] -> w8
    tunnel: [w739] -> _
    tunnel: [w738] -> _
    stop <- w738 stop-if-true
    w737 = 500  # Should not be -1, or do not quit as subVI
    n196 = event shown="[0] Timeout" {
      selector: _ -> [_ _ _ _ _ _ _ _ _ _ _ _ _ _ _]
      dyn-events: _ -> [_ _ _ _ _ _ _ _ _ _ _ _ _ _ _]
      timeout: w737 -> [_ _ _ _ _ _ _ _ _ _ _ _ _ _ _]
      tunnel: w744 -> [w755 w771 w775 w779 w784 w786 w794 w796 w798 w800 w802 w804 w806 w808 w810]
      tunnel: w743 -> [_ _ _ _ w781 _ _ _ _ _ _ _ _ _ _]
      tunnel: w742 -> [w754 _ _ _ _ _ _ _ _ _ _ _ _ _ _]
      tunnel: [_ _ _ _ _ _ TRUE _ _ _ _ _ _ _ _] -> w739
      tunnel: [w753 _ _ _ _ _ errorcluster {"status"=FALSE, "code"=0, "source"=""} ("error constant") _ _ _ _ _ _ _ _] -> w740
      tunnel: w737 -> [w745 _ _ _ _ _ _ _ _ _ _ _ _ _ _]
      event Timeout {
        n197 = event-data() -> ()  [unwired: 1 in, 1 out]
        n198 = Bundle By Name(cluster=T8 {"GenericDAQ State"=enum."GetStat_", "Variant"=variant} ("element"), "Variant"=w754) -> (w751:T8)
        n199 = Enqueue Element At Opposite End "To get LiveStat,\nIt has to be opposite end"(queue=w755, element=w751) -> (error out=w750:errorcluster)  [unwired: 2 in, 2 out]
        n200 = Dequeue Element(queue=w754, timeout in ms (-1)=100, error in (no error)=w750) -> (element=w749:T1, timed out?=w747:bool, error out=w753:errorcluster)  [unwired: 1 out]
        n201 = case shown="False" w747 {
          tunnel: w749 -> [w764 w767]
          tunnel: [w763 w766] -> w748
          tunnel: w745 -> [w759 _]
          frame False {
            n202 = Unbundle By Name(w764) -> ("TrigCount"=w762:i32)
            n203 = feedback-in #1(w762) -> ()
            n204 = feedback #1(0 ("TrigCount")) -> (w761:i32)
            n205 = Subtract(x=w762, y=w761) -> (x-y=w760:i32)
            n206 = Compound Arithmetic op=MULTIPLY(w760, invert w759, 1000.0 ("value")) -> (w757:dbl)
            n207 = Bundle By Name(cluster=w764, "TrigRate(Hz)"=w757) -> (w763:T1)
          }
          frame True {
            n208 = Bundle By Name(cluster=w767, "Model"="timeout !") -> (w766:T1)
          }
        }
        "LiveStat" <- w748
      }
      event Value Change {
        n209 = event-data() -> ("NewVal"=w768:T12)  [unwired: 1 in]
        n210 = Bundle By Name(cluster=T8 {"GenericDAQ State"=enum."SetAcquisition_", "Variant"=variant} ("element"), "Variant"=w768) -> (w769:T8)
        n211 = Enqueue Element(queue=w771, element=w769) -> ()  [unwired: 2 in, 3 out]
      }
      event Value Change {
        n212 = event-data() -> ("NewVal"=w772:cluster{"Range":u32, "DC Offset":i32}[])  [unwired: 1 in]
        n213 = Bundle By Name(cluster=T8 {"GenericDAQ State"=enum."SetChannels_", "Variant"=variant} ("element"), "Variant"=w772) -> (w773:T8)
        n214 = Enqueue Element(queue=w775, element=w773) -> ()  [unwired: 2 in, 3 out]
      }
      event Value Change {
        n215 = event-data() -> ("NewVal"=w776:T7)  [unwired: 1 in]
        n216 = Bundle By Name(cluster=T8 {"GenericDAQ State"=enum."SetTrigger_", "Variant"=variant} ("element"), "Variant"=w776) -> (w777:T8)
        n217 = Enqueue Element(queue=w779, element=w777) -> ()  [unwired: 2 in, 3 out]
      }
      event "ConfigAll": Value Change {
        n218 = event-data() -> ()  [unwired: 1 in, 1 out]
        n219 = property class="Clust (strict)"(reference=w781) -> ("Value"=w780:T3)  [unwired: 1 in, 2 out]
        n220 = Bundle By Name(cluster=T8 {"GenericDAQ State"=enum."SetAll_AcquChTrig_", "Variant"=variant} ("element"), "Variant"=w780) -> (w782:T8)
        n221 = Enqueue Element(queue=w784, element=w782) -> ()  [unwired: 2 in, 3 out]
      }
      event "Get_ConfigAll": Value Change {
        n222 = event-data() -> ()  [unwired: 1 in, 1 out]
        n223 = for {
          tunnel: w786 -> [w790]
          shift-right: [w789] -> _
          shift-left: _ -> [w788]
          tunnel: T8[] [{"GenericDAQ State"=enum."GetAcquisition", "Variant"=variant}, {"GenericDAQ State"=enum."GetChannels", "Variant"=variant}, {"GenericDAQ State"=enum."GetTrigger", "Variant"=variant}] -> [w787] mode=indexing
          n224 = Enqueue Element(queue=w790, element=w787, error in (no error)=w788) -> (error out=w789:errorcluster)  [unwired: 1 in, 2 out]
        }
      }
      event "Quit": Value Change {
        n225 = event-data() -> ()  [unwired: 1 in, 1 out]
        n226 = Enqueue Element(queue=w794, element=T8 {"GenericDAQ State"=enum."Quit", "Variant"=variant}) -> ()  [unwired: 2 in, 3 out]
      }
      event "fConfig": Value Change {
        n227 = event-data() -> ()  [unwired: 1 in, 1 out]
        n228 = Enqueue Element(queue=w796, element=T8 {"GenericDAQ State"=enum."fConfigurate", "Variant"=variant}) -> ()  [unwired: 2 in, 3 out]
      }
      event "Start": Value Change {
        n229 = event-data() -> ()  [unwired: 1 in, 1 out]
        n230 = Enqueue Element(queue=w798, element=T8 {"GenericDAQ State"=enum."fStart", "Variant"=variant}) -> ()  [unwired: 2 in, 3 out]
      }
      event "Reset": Value Change {
        n231 = event-data() -> ()  [unwired: 1 in, 1 out]
        n232 = Enqueue Element(queue=w800, element=T8 {"GenericDAQ State"=enum."Reset", "Variant"=variant}) -> ()  [unwired: 2 in, 3 out]
      }
      event "CloseAll": Value Change {
        n233 = event-data() -> ()  [unwired: 1 in, 1 out]
        n234 = Enqueue Element(queue=w802, element=T8 {"GenericDAQ State"=enum."CloseAll", "Variant"=variant}) -> ()  [unwired: 2 in, 3 out]
      }
      event "Close": Value Change {
        n235 = event-data() -> ()  [unwired: 1 in, 1 out]
        n236 = Enqueue Element(queue=w804, element=T8 {"GenericDAQ State"=enum."Close", "Variant"=variant}) -> ()  [unwired: 2 in, 3 out]
      }
      event "Open": Value Change {
        n237 = event-data() -> ()  [unwired: 1 in, 1 out]
        n238 = Enqueue Element(queue=w806, element=T8 {"GenericDAQ State"=enum."Open", "Variant"=variant}) -> ()  [unwired: 2 in, 3 out]
      }
      event "Enumerate": Value Change {
        n239 = event-data() -> ()  [unwired: 1 in, 1 out]
        n240 = Enqueue Element(queue=w808, element=T8 {"GenericDAQ State"=enum."Enumerate", "Variant"=variant}) -> ()  [unwired: 2 in, 3 out]
      }
      event "StartAll": Value Change {
        n241 = event-data() -> ()  [unwired: 1 in, 1 out]
        n242 = property on="GenericDAQ_Config" class="Clust (strict)"() -> ("Value"=w809:T3)  [unwired: 2 in, 2 out]
        n243 = Bundle By Name(cluster=T8 {"GenericDAQ State"=enum."SetAll_AcquChTrig_", "Variant"=variant} ("element"), "Variant"=w809) -> (w814:T8)
        n244 = Build Array(T8 {"GenericDAQ State"=enum."Enumerate", "Variant"=variant} ("element"), T8 {"GenericDAQ State"=enum."Open", "Variant"=variant} ("element"), w814, T8 {"GenericDAQ State"=enum."fConfigurate", "Variant"=variant} ("element"), T8 {"GenericDAQ State"=enum."fStart", "Variant"=variant} ("element")) -> (w817:T8[])
        n245 = for {
          shift-right: [w821] -> _
          shift-left: w810 -> [w822]
          tunnel: w817 -> [w820] mode=indexing
          shift-right: [w819] -> _
          shift-left: _ -> [w818]
          n246 = Enqueue Element(queue=w822, element=w820, error in (no error)=w818) -> (queue out=w821:refnum<queue>, error out=w819:errorcluster)  [unwired: 1 in, 1 out]
        }
      }
    }
    n247 = Or(x=w739, y=w741) -> (x .or. y?=w738:bool)
  }
  n248 = Release Queue(queue=w17, error in (no error)=w15) -> (error out=w21:errorcluster)  [unwired: 1 in, 2 out]
  n249 = Release Queue(queue=w22, error in (no error)=w21) -> (error out=w19:errorcluster)  [unwired: 1 in, 2 out]
  n250 = Merge Errors(w8, w19) -> (w9:errorcluster)
  n251 = Release Queue(queue=w20, error in (no error)=w9) -> (error out=w14:errorcluster)  [unwired: 1 in, 2 out]
  n252 = call <vilib>:"General Error Handler.vi"("type of dialog (OK msg:1)"=w13, "error in (no error)"=w14, "[exception action] (none:0)"=w12, "[exception code]"=w11) -> ()  [unwired: 7 in, 5 out]
